vi "FilterOverlappedDroplets.vi"(8 "error in (no error)":errorcluster, 9 "Circle Descriptor":cluster{"Min Radius":dbl, "Max Radius":dbl}={"Min Radius"=3.0, "Max Radius"=500.0}, 10 "Threshold (pixels)":dbl, 11 "Circles (Calibrated)":T1(array[cluster]) {"Position"."Y" format="%.2f"; "Position"."X" format="%.2f"}) -> (0 "error out":errorcluster, 3 "Circles (Calibrated) 2":T1(array[cluster]) {"Position"."Y" format="%.2f"; "Position"."X" format="%.2f"})   [LabVIEW 2013]
doc: "Use this template to build a VI to use as a subVI."
panel:
  out "Input Array Size":i32
  out "Output Array size":i32
  out "size(s)":i32
  out "Array":cluster{"index of element":i32, i32}[](array[cluster])
  out "Found overlapping Droplet":bool[][](array[boolean])
  out "Distance Matrix":sgl[][](array[numeric])
  # "Filters out droplets that apear one on top of the other and grabs the larger of the two."
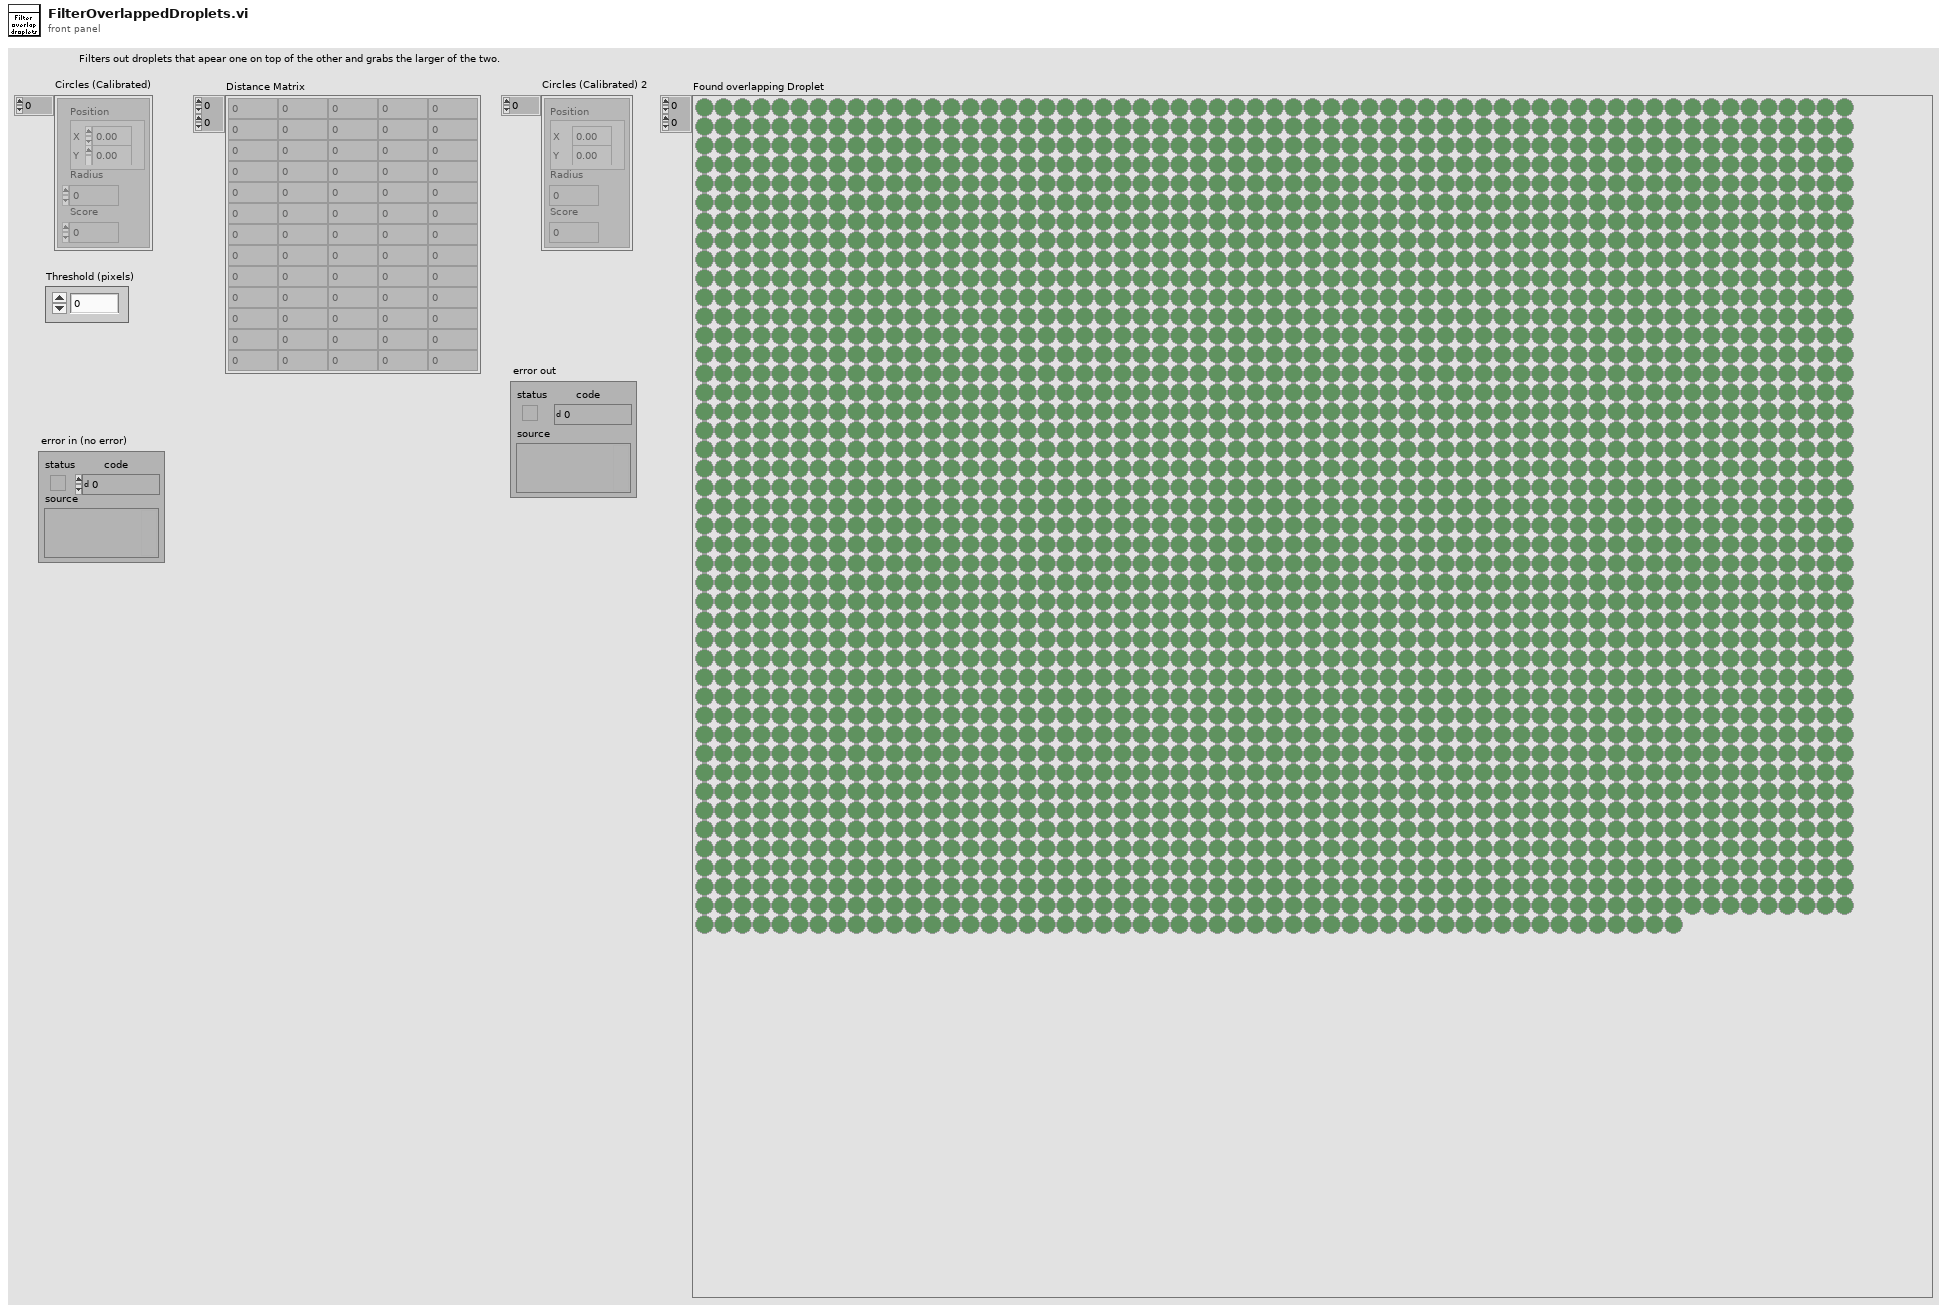
[diagram p1: front panel]
types:
  T1 = cluster{"Position":cluster{"X":sgl, "Y":sgl}, "Radius":dbl, "Score":dbl}[]
  T2 = cluster{"Position":cluster{"X":sgl, "Y":sgl}, "Radius":dbl, "Score":dbl}
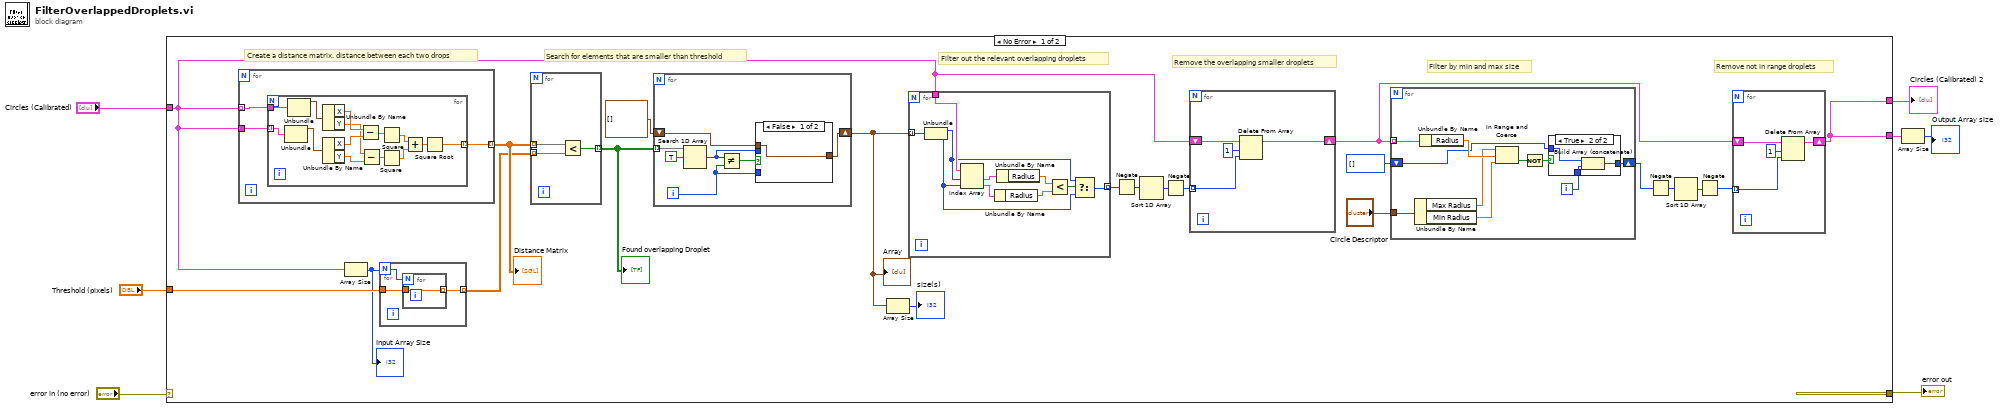
[diagram p0: block diagram]
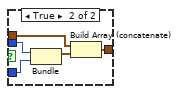
[diagram p3: hidden frame]
diagram:
  n1 = case shown="No Error" "error in (no error)" {
    selector: "error in (no error)" -> [_ w98]
    tunnel: [_ w98] -> w6
    tunnel: "Circles (Calibrated)" -> [w20 _]
    tunnel: "Threshold (pixels)" -> [w27 _]
    tunnel: [w12 _] -> w2
    tunnel: [w12 _] -> w1
    frame No Error {
      # "Remove not in range droplets"
      # "Filter by min and max size"
      # "Remove the overlapping smaller droplets"
      # "Filter out the relevant overlapping droplets"
      # "Search for elements that are smaller than threshold"
      # "Create a distance matrix. distance between each two drops"
      n2 = for {
        tunnel: w20 -> [w82] mode=indexing
        tunnel: w20 -> [w83]
        tunnel: [w81] -> w28 mode=indexing
        n3 = for {
          tunnel: w83 -> [w95] mode=indexing
          tunnel: w82 -> [w96]
          tunnel: [w84] -> w81 mode=indexing
          n4 = Unbundle(w95) -> ("Position"=w94:cluster{"X":sgl, "Y":sgl})  [unwired: 2 out]
          n5 = Unbundle(w96) -> ("Position"=w97:cluster{"X":sgl, "Y":sgl})  [unwired: 2 out]
          n6 = Unbundle By Name(w97) -> ("X"=w93:sgl, "Y"=w90:sgl)
          n7 = Unbundle By Name(w94) -> ("X"=w92:sgl, "Y"=w89:sgl)
          n8 = Subtract(x=w93, y=w92) -> (x-y=w91:sgl)
          n9 = Subtract(x=w90, y=w89) -> (x-y=w88:sgl)
          n10 = Square(x=w88) -> (x^2=w86:sgl)
          n11 = Square(x=w91) -> (x^2=w87:sgl)
          n12 = Add(x=w87, y=w86) -> (x+y=w85:sgl)
          n13 = Square Root(x=w85) -> (sqrt(x)=w84:sgl)
        }
      }
      "Distance Matrix" <- w28
      n14 = Array Size(array=w20) -> (size(s)=w26:i32)
      "Input Array Size" <- w26
      n15 = for {
        N: w26 -> [w75]
        tunnel: w27 -> [w76]
        tunnel: [w74] -> w25 mode=indexing
        n16 = for {
          N: w75 -> [_]
          tunnel: w76 -> [w77]
          tunnel: [w77] -> w74 mode=indexing
        }
      }
      n17 = for {
        tunnel: w28 -> [w80] mode=indexing
        tunnel: w25 -> [w79] mode=indexing
        tunnel: [w78] -> w24 mode=indexing
        n18 = Less?(x=w80, y=w79) -> (x < y?=w78:bool[])
      }
      "Found overlapping Droplet" <- w24
      n19 = for {
        tunnel: w24 -> [w67] mode=indexing
        shift-right: [w61] -> w21
        shift-left: cluster{"index of element":i32, i32}[] [] -> [w62]
        i -> [w63]
        n20 = Search 1D Array(1D array=w67, element=TRUE) -> (index of element=w64:i32)  [unwired: 1 in]
        n21 = Not Equal?(x=w64, y=w63) -> (x != y?=w65:bool)
        n22 = case shown="False" w65 {
          tunnel: w64 -> [_ w72]
          tunnel: w63 -> [_ w73]
          tunnel: [w68 w71] -> w61
          tunnel: w62 -> [w68 w70]
          frame False {
          }
          frame True {
            n23 = Bundle("index of element"=w72, w73) -> (w69:cluster{"index of element":i32, i32})  [unwired: 1 in]
            n24 = Build Array (concatenate)(w70, w69) -> (w71:cluster{"index of element":i32, i32}[])
          }
        }
      }
      "Array" <- w21
      n25 = Array Size(array=w21) -> (size(s)=→"size(s)":i32)
      n26 = for {
        tunnel: w21 -> [w60] mode=indexing
        tunnel: w20 -> [w59]
        tunnel: [w53] -> w17 mode=indexing
        n27 = Unbundle(w60) -> ("index of element"=w55:i32, w54:i32)
        n28 = Index Array(array=w59, index #1=w55, index #2=w54) -> (element #1=w52:T2, element #2=w58:T2)
        n29 = Unbundle By Name(w58) -> ("Radius"=w57:dbl)
        n30 = Unbundle By Name(w52) -> ("Radius"=w51:dbl)
        n31 = Less?(x=w51, y=w57) -> (x < y?=w56:bool)
        n32 = Select(t=w55, s=w56, f=w54) -> (s? t:f=w53:i32)
      }
      n33 = Negate(x=w17) -> (-x=w16:i32[])
      n34 = Sort 1D Array(array=w16) -> (sorted array=w19:i32[])
      n35 = Negate(x=w19) -> (-x=w18:i32[])
      n36 = for {
        shift-right: [w48] -> w13
        shift-left: w20 -> [w49]
        tunnel: w18 -> [w47] mode=indexing
        n37 = Delete From Array(array=w49, length=1, index=w47) -> (array with subset deleted=w48:T1)  [unwired: 1 out]
      }
      n38 = for {
        tunnel: "Circle Descriptor" -> [w42]
        tunnel: w13 -> [w41] mode=indexing
        shift-right: [w34] -> w9
        shift-left: i32[] [] -> [w33]
        i -> [w35]
        n39 = Unbundle By Name(w42) -> ("Max Radius"=w39:dbl, "Min Radius"=w38:dbl)
        n40 = Unbundle By Name(w41) -> ("Radius"=w40:dbl)
        n41 = In Range and Coerce(upper limit=w39, x=w40, lower limit=w38) -> (In Range?=w37:bool)  [unwired: 1 out]
        n42 = Not(x=w37) -> (.not. x?=w36:bool)
        n43 = case shown="True" w36 {
          tunnel: w35 -> [_ w46]
          tunnel: [w43 w45] -> w34
          tunnel: w33 -> [w43 w44]
          frame False {
          }
          frame True {
            n44 = Build Array (concatenate)(w44, w46) -> (w45:i32[])
          }
        }
      }
      n45 = Negate(x=w9) -> (-x=w11:i32[])
      n46 = Sort 1D Array(array=w11) -> (sorted array=w10:i32[])
      n47 = Negate(x=w10) -> (-x=w8:i32[])
      n48 = for {
        shift-right: [w30] -> w12
        shift-left: w13 -> [w31]
        tunnel: w8 -> [w29] mode=indexing
        n49 = Delete From Array(array=w31, length=1, index=w29) -> (array with subset deleted=w30:T1)  [unwired: 1 out]
      }
    }
    frame Error {
    }
  }
  "error out" <- w6
  "Circles (Calibrated) 2" <- w2
  n50 = Array Size(array=w1) -> (size(s)=→"Output Array size":i32)
